vi "PENDIENTE DE UNA RECTA.vi"() -> ()   [LabVIEW 2020]
panel:
  in  "stop":bool
  out "CRUCE POR CERO":dbl
  out "\"m\"":dbl
  in  "Y2":dbl
  in  "Y1":dbl
  in  "X2":dbl
  in  "X1":dbl
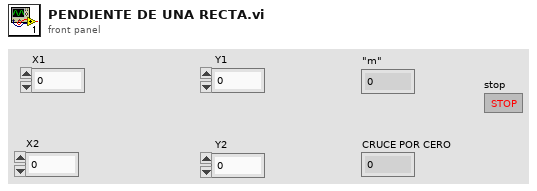
[diagram p1: front panel]
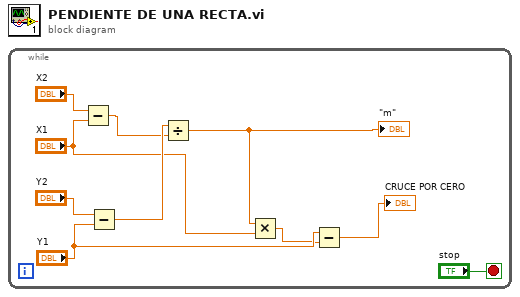
[diagram p0: block diagram]
diagram:
  n1 = while {
    stop <- "stop" stop-if-true
    n2 = Subtract(x="X2", y="X1") -> (x-y=w7:dbl)
    n3 = Subtract(x="Y2", y="Y1") -> (x-y=w8:dbl)
    n4 = Divide(x=w8, y=w7) -> (x/y=w6:dbl)
    "\"m\"" <- w6
    n5 = Multiply(x=w6, y="X1") -> (x*y=w3:dbl)
    n6 = Subtract(x="Y1", y=w3) -> (x-y=→"CRUCE POR CERO":dbl)
  }
